vi "MListbox Set Column Header.vi"(5 "Font Color":u32(colorbox), 6 "Active Cell:Cell Font:Bold":bool, 7 "Font:Size":u32=20, 8 "error in (no error)":errorcluster, 9 "Justification":enum16{"Left", "Center", "Right"}(ring), 10 "Column Headers":string[](array[string]), 11 "Multicolumn ListBox in":refnum<class "Multicolumn ListBox.lvclass">) -> (0 "error out":errorcluster, 3 "Multicolumn ListBox out":refnum<class "Multicolumn ListBox.lvclass">)   [LabVIEW 2018, in "Multicolumn ListBox.lvclass"]
uses:
  Multicolumn ListBox.lvclass
  <vilib>/Utility/miscctls.llb/LVRowAndColumnTypeDef.ctl
  Multicolumn ListBox.lvclass/Multicolumn ListBox.ctl
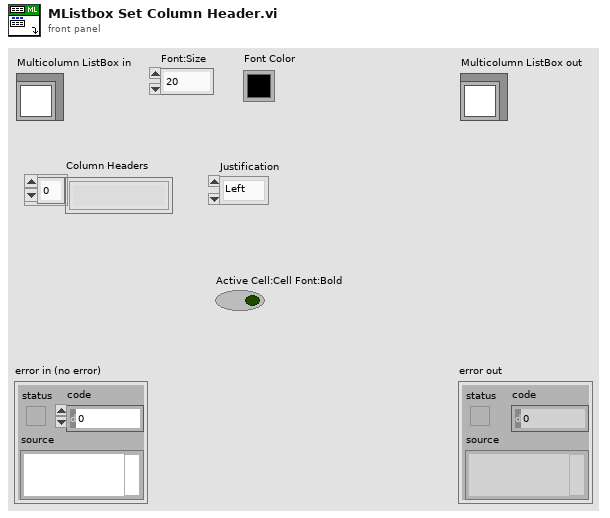
[diagram p1: front panel]
types:
  T1 = typedef "LVRowAndColumnTypeDef.ctl" = cluster{"Row":i32, "Column":i32}
  T2 = cluster{"left":i16, "top":i16, "right":i16, "bottom":i16}
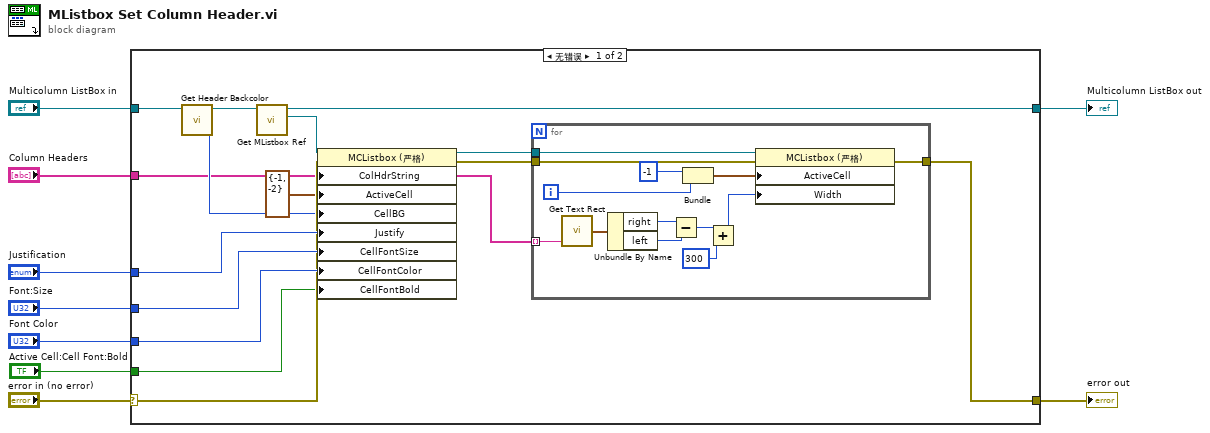
[diagram p0: block diagram]
diagram:
  n1 = case shown="无错误" "error in (no error)" {
    selector: "error in (no error)" -> [w18 w39]
    tunnel: [w11 w39] -> w8
    tunnel: [w23 w38] -> w6
    tunnel: "Multicolumn ListBox in" -> [w24 w38]
    tunnel: "Column Headers" -> [w14 _]
    tunnel: "Justification" -> [w21 _]
    tunnel: "Font:Size" -> [w20 _]
    tunnel: "Font Color" -> [w19 _]
    tunnel: "Active Cell:Cell Font:Bold" -> [w10 _]
    frame No Error {
      n2 = call "Get Header Backcolor.vi"("Multicolumn ListBox in"=w24) -> ("Header Backcolor"=w16:u32, "Multicolumn ListBox out"=w17:refnum<class "Multicolumn ListBox.lvclass">)  [unwired: 8 in, 1 out]
      n3 = call "Get MListbox Ref.vi"("Multicolumn ListBox in"=w17) -> ("MListbox Ref"=w22:refnum<vi>, "Multicolumn ListBox out"=w23:refnum<class "Multicolumn ListBox.lvclass">)  [unwired: 8 in, 1 out]
      n4 = property class="MCListbox (严格)"(reference=w22, error in=w18, "ColHdrString"=w14, "ActiveCell"=T1 {"Row"=-1, "Column"=-2} ("Active Cell:Active Cell"), "CellBG"=w16, "Justify"=w21, "CellFontSize"=w20, "CellFontColor"=w19, "CellFontBold"=w10) -> (reference out=w13:refnum<vi>, error out=w12:errorcluster)
      n5 = for {
        tunnel: w14 -> [w37] mode=indexing
        tunnel: w13 -> [w33]
        tunnel: w12 -> [w32]
        tunnel: [w25] -> w11
        i -> [w27]
        n6 = call <vilib>:"Get Text Rect.vi"("text"=w37) -> ("rect"=w36:T2)  [unwired: 8 in]
        n7 = Unbundle By Name(w36) -> ("right"=w35:i16, "left"=w34:i16)
        n8 = Subtract(x=w35, y=w34) -> (x-y=w31:i16)
        n9 = Bundle("Row"=-1, w27) -> (w26:cluster{"Row":i32, i32})  [unwired: 1 in]
        n10 = Add(x=w31, y=300) -> (x+y=w29:i32)
        n11 = property class="MCListbox (严格)"(reference=w33, error in=w32, "ActiveCell"=w26, "Width"=w29) -> (error out=w25:errorcluster)  [unwired: 1 out]
      }
    }
    frame Error {
    }
  }
  "error out" <- w8
  "Multicolumn ListBox out" <- w6
